vi "sense.vi"(2 "Y":i8, 3 "X":i8, 4 "World":i8[][](array[numeric])) -> (0 "Heading":i8, 1 "Sensor Array":i8[][](array[numeric]))   [LabVIEW 2012]
doc: "This VI returns a 3x3 subsection of the world array and the direction of the highest-valued neighbor based on the Vcode key. If there is no highest-valued neighbor, it returns a random number from 1 to 8."
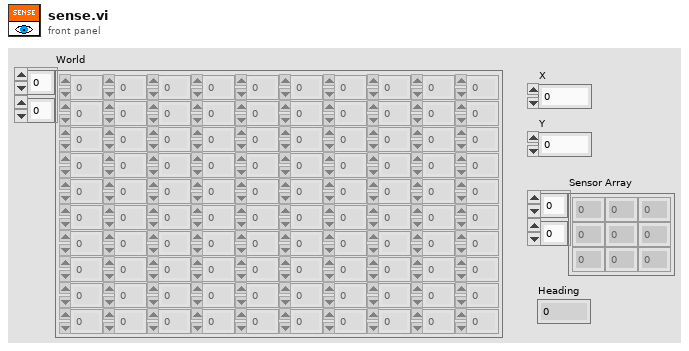
[diagram p1: front panel]
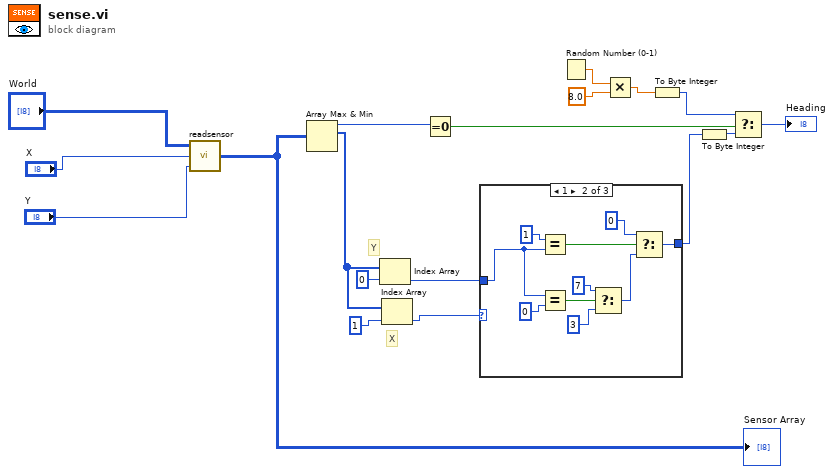
[diagram p0: block diagram]
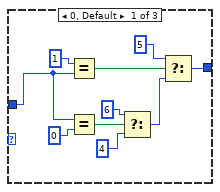
[diagram p2: hidden frame]
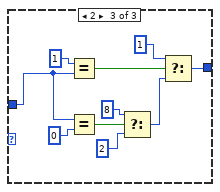
[diagram p3: hidden frame]
diagram:
  # "X"
  # "Y"
  n1 = call "readsensor.vi"("Y"="Y", "X"="X", "World"="World") -> ("Sensor Array"=w15:i8[][])
  "Sensor Array" <- w15
  n2 = Array Max & Min(array=w15) -> (max value=w14:i8, max index (indices)=w6:i32[])  [unwired: 2 out]
  n3 = Index Array(array=w6, index=0) -> (element=w3:i32)
  n4 = Index Array(array=w6, index=1) -> (element=w7:i32)
  n5 = Equal To 0?(x=w14) -> (x = 0?=w8:bool)
  n6 = case shown="1" w7 {
    tunnel: w3 -> [w23 w33 w43]
    tunnel: [w28 w38 w48] -> w1
    frame 0, Default {
      n7 = Equal?(x=1, y=w23) -> (x = y?=w27:bool)
      n8 = Equal?(x=w23, y=0) -> (x = y?=w24:bool)
      n9 = Select(t=6, s=w24, f=4) -> (s? t:f=w26:i32)
      n10 = Select(t=5, s=w27, f=w26) -> (s? t:f=w28:i32)
    }
    frame 1 {
      n11 = Equal?(x=1, y=w33) -> (x = y?=w37:bool)
      n12 = Equal?(x=w33, y=0) -> (x = y?=w34:bool)
      n13 = Select(t=7, s=w34, f=3) -> (s? t:f=w36:i32)
      n14 = Select(t=0, s=w37, f=w36) -> (s? t:f=w38:i32)
    }
    frame 2 {
      n15 = Equal?(x=1, y=w43) -> (x = y?=w47:bool)
      n16 = Equal?(x=w43, y=0) -> (x = y?=w44:bool)
      n17 = Select(t=8, s=w44, f=2) -> (s? t:f=w46:i32)
      n18 = Select(t=1, s=w47, f=w46) -> (s? t:f=w48:i32)
    }
  }
  n19 = Random Number (0-1)() -> (number: 0 to 1=w10:dbl)
  n20 = Multiply(x=w10, y=8.0) -> (x*y=w11:dbl)
  n21 = To Byte Integer(number=w11) -> (8bit integer=w12:i8)
  n22 = To Byte Integer(number=w1) -> (8bit integer=w2:i8)
  n23 = Select(t=w12, s=w8, f=w2) -> (s? t:f=→"Heading":i8)
